vi "subTimeOut.vi"(10 "Timeout (sec)":dbl, 11 "Arduino Resource":T1={"VISA resource"="", "Board Type"=enum."Uno", "Connection Type"=enum."USB / Serial", "Bytes Per Packet (15)"=15}) -> (3 "Arduino Resource 2":T1={"VISA resource"="", "Board Type"=enum."Uno", "Connection Type"=enum."USB / Serial", "Bytes Per Packet (15)"=15})   [LabVIEW 2016]
uses:
  <vilib>/LabVIEW Interface for Arduino/Type Defs/Arduino Resource.ctl
  <vilib>/LabVIEW Interface for Arduino/Type Defs/Board Type.ctl
  <vilib>/LabVIEW Interface for Arduino/LabVIEW Interface for Arduino.lvlib
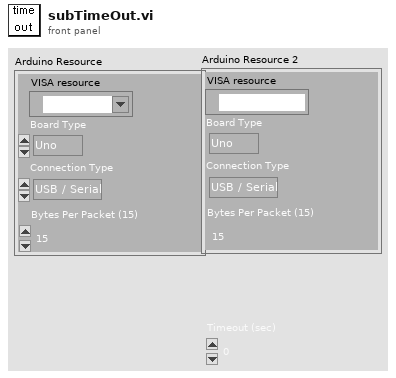
[diagram p1: front panel]
types:
  T1 = typedef "LabVIEW Interface for Arduino.lvlib/Arduino Resource.ctl" = cluster{"VISA resource":refnum<visa-resource-name>, "Board Type":T2, "Connection Type":enum8{"USB / Serial"}, "Bytes Per Packet (15)":u8}
  T2 = typedef "LabVIEW Interface for Arduino.lvlib/Board Type.ctl" = enum16{"Uno", "Dimuelanove w/Atmega 328", "Mega 2560"}
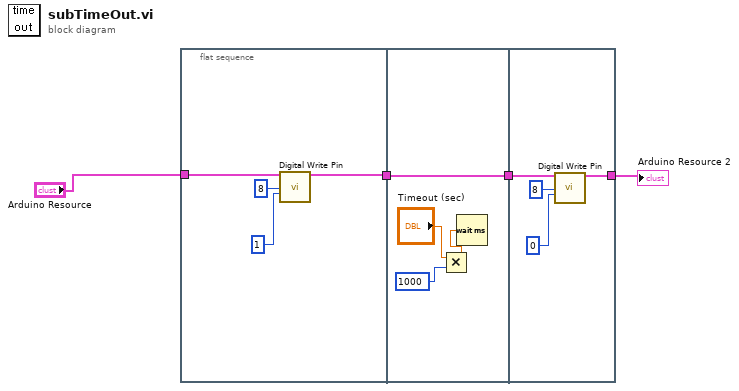
[diagram p0: block diagram]
diagram:
  n1 = flat-sequence {
    tunnel: "Arduino Resource" -> [w6]
    tunnel: [w5] -> w2
    tunnel: w2 -> [w12]
    tunnel: [w12] -> w1
    tunnel: [w13] -> w3
    tunnel: w1 -> [w14]
    frame #0 {
      n2 = call <vilib>:"Digital Write Pin.vi"("Arduino Resource"=w6, "Digital I/O Pin (0)"=8, "Value (0)"=1) -> ("Arduino Resource"=w5:T1)  [unwired: 11 in, 1 out]
    }
    frame #1 {
      n3 = Multiply(x="Timeout (sec)", y=1000) -> (x*y=w11:dbl)
      n4 = Wait (ms)(milliseconds to wait=w11) -> ()  [unwired: 1 out]
    }
    frame #2 {
      n5 = call <vilib>:"Digital Write Pin.vi"("Arduino Resource"=w14, "Digital I/O Pin (0)"=8, "Value (0)"=0) -> ("Arduino Resource"=w13:T1)  [unwired: 11 in, 1 out]
    }
  }
  "Arduino Resource 2" <- w3
